vi "NewPower_Range.vi"(10 "电流值":dbl) -> (0 "switch":bool[](array[boolean]), 1 "current":dbl, 2 "region":string, 3 "adress":string)   [LabVIEW 2015]
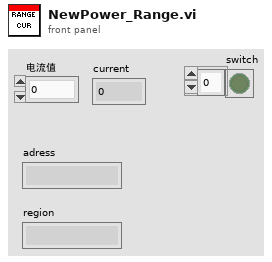
[diagram p1: front panel]
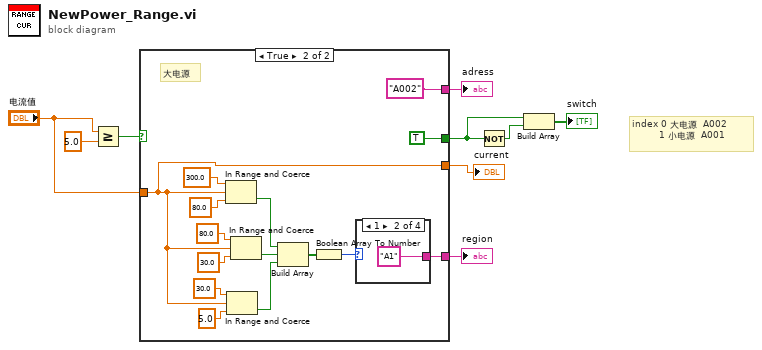
[diagram p0: block diagram]
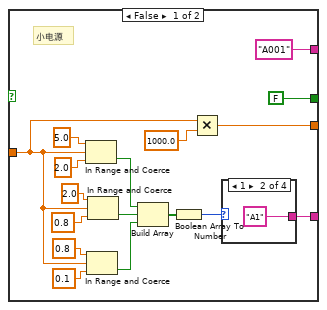
[diagram p2: hidden frame]
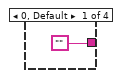
[diagram p3: hidden frame]
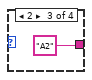
[diagram p4: hidden frame]
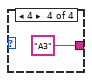
[diagram p5: hidden frame]
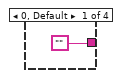
[diagram p6: hidden frame]
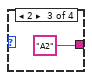
[diagram p7: hidden frame]
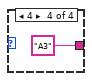
[diagram p8: hidden frame]
diagram:
  # "index 0 大电源  A002\n         1 小电源  A001"
  n1 = Greater Or Equal?(x="电流值", y=5.0) -> (x >= y?=w7:bool)
  n2 = case shown="True" w7 {
    tunnel: ["A001" ("format string") "A002" ("format string")] -> w5
    tunnel: [FALSE TRUE] -> w1
    tunnel: "电流值" -> [w12 w31]
    tunnel: [w13 w32] -> w4
    tunnel: [w10 w31] -> w3
    frame False {
      # "小电源"
      n3 = In Range and Coerce(upper limit=5.0, x=w12, lower limit=2.0) -> (In Range?=w18:bool)  [unwired: 1 out]
      n4 = In Range and Coerce(upper limit=0.8, x=w12, lower limit=0.1) -> (In Range?=w16:bool)  [unwired: 1 out]
      n5 = In Range and Coerce(upper limit=2.0, x=w12, lower limit=0.8) -> (In Range?=w17:bool)  [unwired: 1 out]
      n6 = Build Array(w18, w17, w16) -> (w15:bool[])
      n7 = Boolean Array To Number(Boolean array=w15) -> (number=w14:u32)
      n8 = Multiply(x=w12, y=1000.0) -> (x*y=w10:dbl)
      n9 = case shown="1" w14 {
        tunnel: ["" "A1" ("format string") "A2" ("format string") "A3" ("format string")] -> w13
        frame 0, Default {
        }
        frame 1 {
        }
        frame 2 {
        }
        frame 4 {
        }
      }
    }
    frame True {
      # "大电源"
      n10 = In Range and Coerce(upper limit=300.0, x=w31, lower limit=80.0) -> (In Range?=w38:bool)  [unwired: 1 out]
      n11 = In Range and Coerce(upper limit=30.0, x=w31, lower limit=5.0) -> (In Range?=w36:bool)  [unwired: 1 out]
      n12 = In Range and Coerce(upper limit=80.0, x=w31, lower limit=30.0) -> (In Range?=w37:bool)  [unwired: 1 out]
      n13 = Build Array(w38, w37, w36) -> (w35:bool[])
      n14 = Boolean Array To Number(Boolean array=w35) -> (number=w34:u32)
      n15 = case shown="1" w34 {
        tunnel: ["" "A1" ("format string") "A2" ("format string") "A3" ("format string")] -> w32
        frame 0, Default {
        }
        frame 1 {
        }
        frame 2 {
        }
        frame 4 {
        }
      }
    }
  }
  "adress" <- w5
  "region" <- w4
  "current" <- w3
  n16 = Not(x=w1) -> (.not. x?=w2:bool)
  n17 = Build Array(w1, w2) -> (→"switch":bool[])
